vi "Create.vi"(8 "error in (no error)":errorcluster, 10 "Run VI":T1, 11 "Job Description":string) -> (0 "error out":errorcluster, 3 "Run VI out":refnum<class "Run VI.lvclass">)   [LabVIEW 2014, in "Run VI.lvclass"]
uses:
  Run VI.lvclass
  Shared/Controls/Run VI - STYP.ctl
  Build Job/Build Job.lvclass/Build Job.ctl
  Run VI.lvclass/Run VI.ctl
  Build Job/Write Script Job Name.vi
  Build Job/Write Job Description.vi
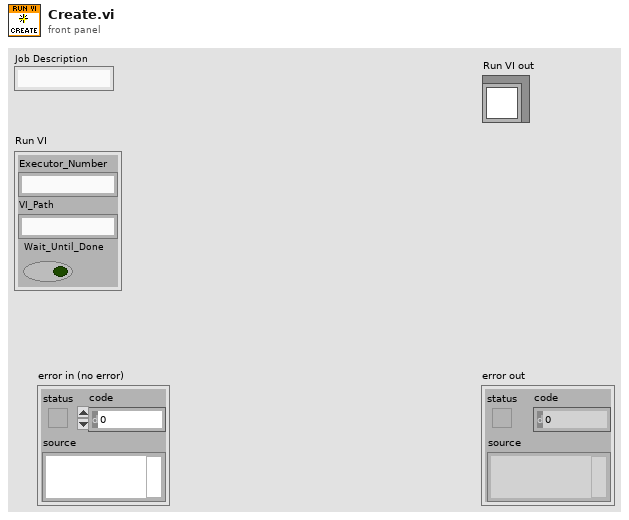
[diagram p1: front panel]
types:
  T1 = typedef "Run VI - STYP.ctl" = cluster{"Executor_Number":string, "VI_Path":string, "Wait_Until_Done":bool}
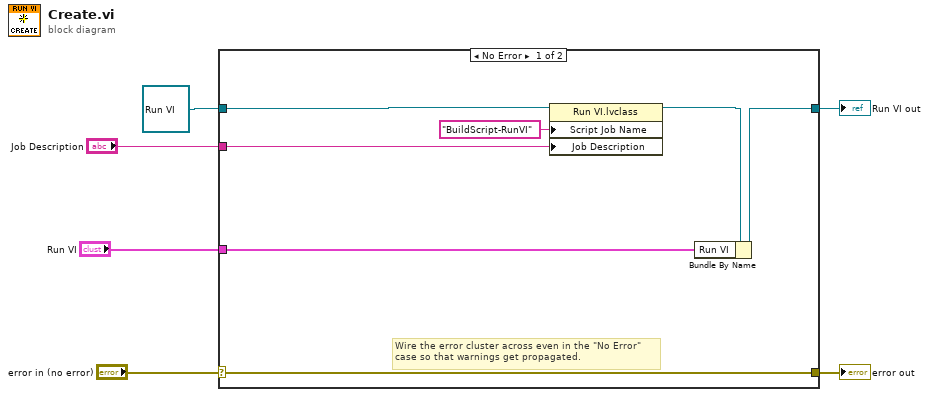
[diagram p0: block diagram]
diagram:
  n1 = case shown="No Error" "error in (no error)" {
    selector: "error in (no error)" -> [w13 w15]
    tunnel: [w13 w15] -> w5
    tunnel: [w7 w14] -> w3
    tunnel: refnum<class "Run VI.lvclass"> refnum ("Run VI in") -> [w12 w14]
    tunnel: "Job Description" -> [w10 _]
    tunnel: "Run VI" -> [w9 _]
    frame No Error {
      # "Wire the error cluster across even in the \"No Error\"\ncase so that warnings get propagated."
      n2 = property class="Run VI.lvclass"(reference=w12, "Script Job Name"="BuildScript-RunVI", "Job Description"=w10) -> (reference out=w8:refnum<class "Run VI.lvclass">)  [unwired: 1 in, 1 out]
      n3 = Bundle By Name(cluster=w8, "Run VI"=w9) -> (w7:refnum<class "Run VI.lvclass">)
    }
    frame Error {
    }
  }
  "error out" <- w5
  "Run VI out" <- w3
